vi "PD_Target.vi"   [LabVIEW 2022 SP3]
uses:
  <vilib>/rvi/interface/RandomDataEmulation/niFpgaRandomDataHandleErrors.vi
  <vilib>/rvi/DataTransferAndStorage/Container/XNode/niFpgaContainer.xnode
  <vilib>/rvi/interface/RandomDataEmulation/nirviRandomDataFpgaReadWriteTemplate.vi
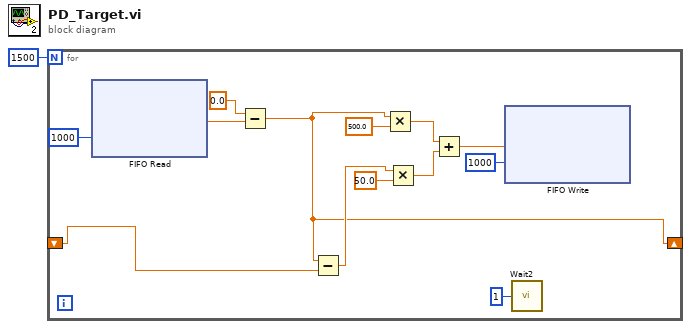
[diagram p0: block diagram]
diagram:
  n1 = for {
    N: 1500 -> [_]
    shift-right: [w2] -> _
    shift-left: _ -> [w3]
    n2 = xnode ("FIFO Read")("Timeout"=1000) -> ("Element"=w5:sgl)  [unwired: 1 in, 2 out]
    n3 = Subtract(x=sgl 0.0, y=w5) -> (x-y=w2:sgl)
    n4 = Subtract(x=w2, y=w3) -> (x-y=w13:sgl)
    n5 = Multiply(x=w2, y=sgl 500.0) -> (x*y=w11:sgl)
    n6 = Multiply(x=w13, y=sgl 50.0) -> (x*y=w10:sgl)
    n7 = Add(x=w11, y=w10) -> (x+y=w9:sgl)
    n8 = xnode ("FIFO Write")("Element"=w9, "Timeout"=1000) -> ()  [unwired: 1 in, 2 out]
    n9 = call "Wait2"("Count(mSec)"=u32 1) -> ()  [unwired: 1 out]
  }
